vi "2022NewInstrumentationU6.vi"() -> ()   [LabVIEW 2021]
uses:
  <vilib>/Analysis/baseanly.llb/Mean (DBL).vi
  <vilib>/Analysis/NI_AALBase.lvlib
panel:
  out "ShuntCurrent":dbl[](graph)
  in  "Clear Charts Button":bool
  out "Runtank Weight":dbl(slide) scale=0.0..5.0
  out "Injector Pressure":dbl(knob) scale=700.0..800.0
  out "Runtank Pressure":dbl(knob) scale=700.0..800.0
  out "N2 Pressure":dbl(knob) scale=700.0..800.0
  out "N20 Pressure":dbl(knob) scale=700.0..800.0
  in  "Binary 2":bool
  in  "AIN Range":u16(ring) items=["LJ_rgBIP10V", "LJ_rgBIP1V", "LJ_rgBIPP1V", "LJ_rgBIPP01V"]
  in  "FirstFound":bool=TRUE
  in  "Address":string="1"
  out "Error Message 2":string="No Error"
  out "error out":errorcluster
  out "Cold Junction Temp":dbl=41420.0 format="%.6f"
  out "L-Thrust":dbl(graph)
  out "L-RunTank":dbl(graph)
  out "P-CombChamb - Deactivated":dbl[](graph)
  out "P-Injector":dbl(graph)
  out "T-PoComb":dbl(graph)
  out "T-CombCham":dbl(graph)
  out "T-Injector":dbl(graph)
  out "T-RunTank":dbl(graph)
  out "P-RunTank":dbl(graph)
  out "P-N2Flow":dbl(graph)
  out "P-N2OFlow":dbl(graph)
  in  "file name":string
  in  "file path":path
  in  "Iterations/Second":i32=1
  in  "Binary":bool
  in  "StreamSettlingFactor":i32
  in  "Resolution Index":u8
  in  "Range Constants":u8[](array[ring])=[0, 0, 0, 0] items=["LJ_rgBIP10V", "LJ_rgBIP1V", "LJ_rgBIPP1V", "LJ_rgBIPP01V"]
  out "Stream Parameters":T1 {"Device Backlog [%]" format="%.2f"}
  in  "PC buffer size (seconds)":dbl=10.0 format="%.2f"
  out "# of iterations":i32
  in  "Scan Rate (Hz)":dbl=1000.0 format="%.3f"
  in  "stop":bool
  out "Error Message":string
  # "Standard Test Parameters:"
  # "Range = 10\nResolution = 3\nSettling Factor = 2\nIterations/Second = 1\nScan Rate = 1300"
  # "This example streams from the first found USB U6."
  # "Data Output For Pressure, Temperature, and Load Sensors"
  # "The + scan list is the positive\nchannels.  For each element in\nthe + list, there must also be\nan element in the - list, which is\nthe negative channels.  For\nsingle-ended channels, put in\n199 for the negative channel.\n\nTo remove an element, right-click\non it, select Data Operations =>\nRemove Element.\n\nTo empty an array, right-click\nnear the edge, select Data\nOperations => Empty Array.\n\nOther useful operations:  From the\nOperate menu are \"Make Current\nValues Default\" and \"Reinitialize\nTo Default\"."
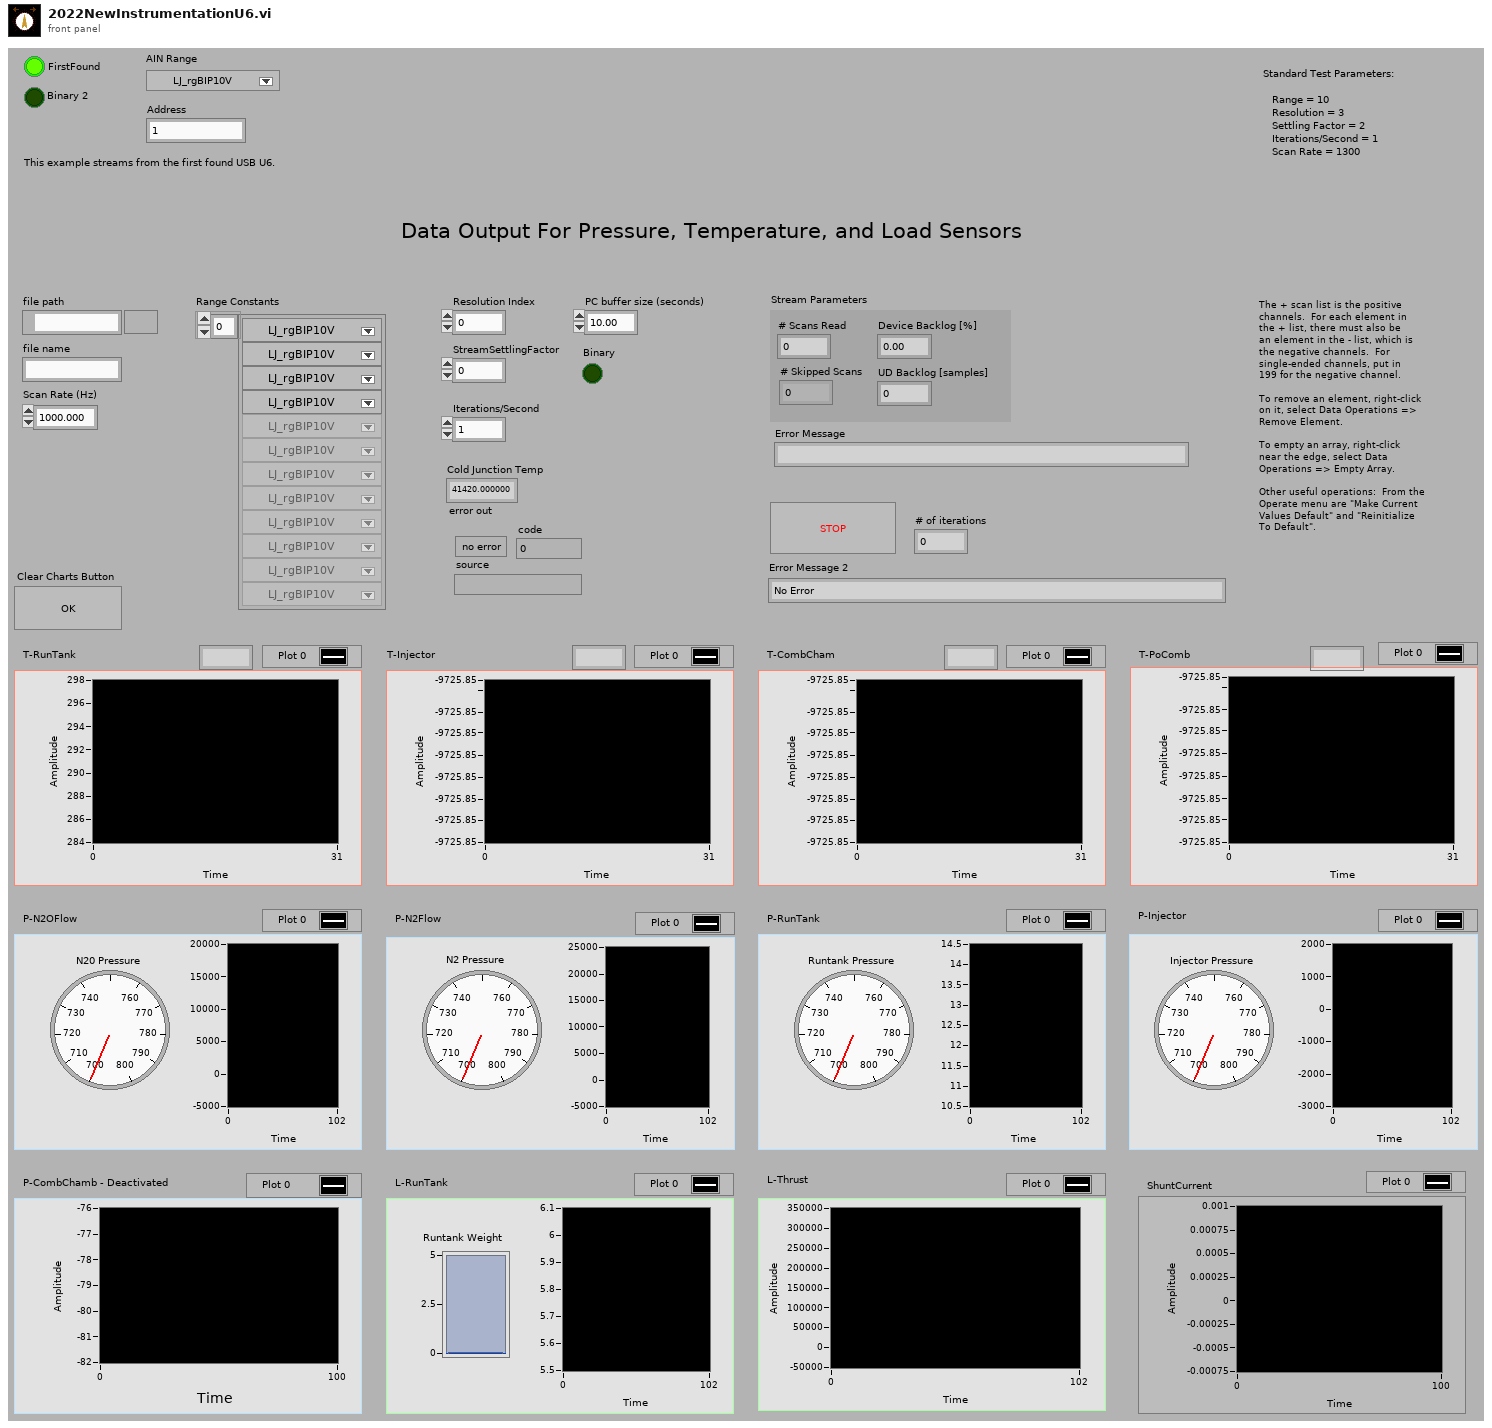
[diagram p1: front panel]
types:
  T1 = cluster{"# Scans Read":i32, "# Skipped Scans":i32, "Device Backlog [%]":dbl, "UD Backlog [samples]":i32}
  T2 = enum16{"open", "open or create", "create or replace", "create", "open (read-only)"}
  T3 = cluster{"PC buffer size (seconds)":dbl, "Resolution Index":u8, "StreamSettlingFactor":i32, "Binary":bool}
  T4 = typedef "Control 1.ctl" = dbl[][]
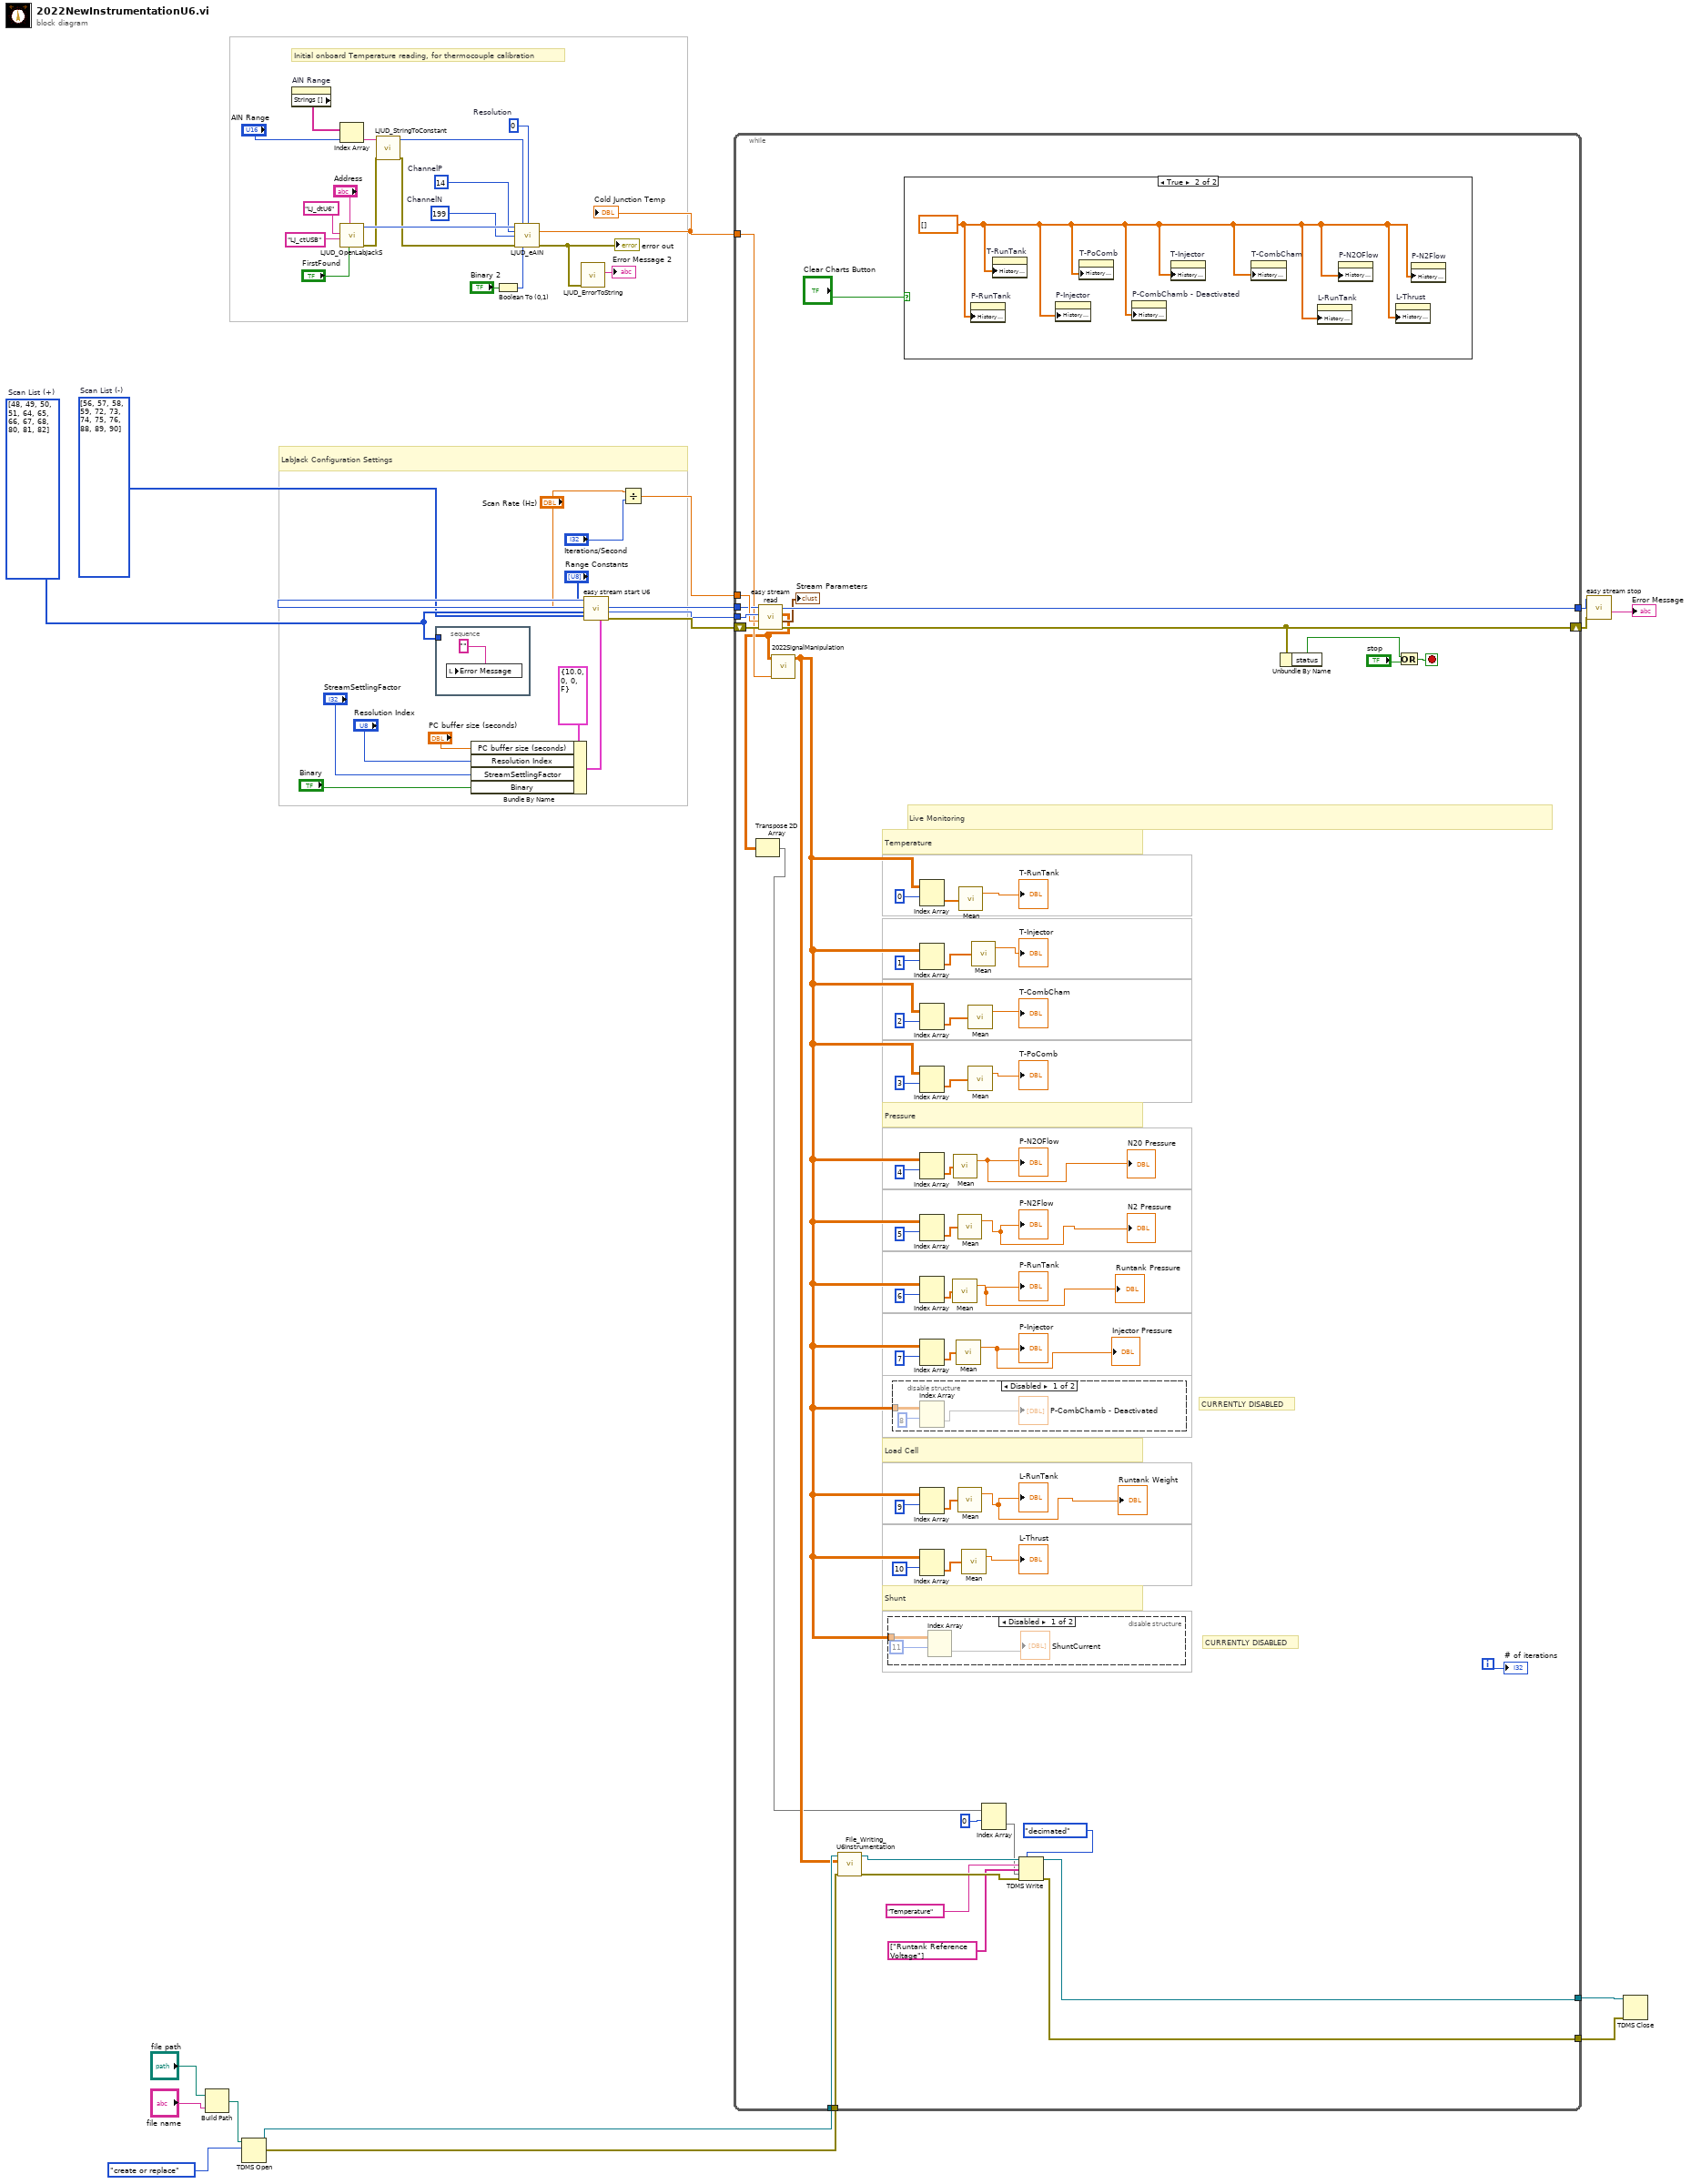
[diagram p0: block diagram]
diagram:
  w20 = 0  # Resolution
  w10 = 199  # ChannelN
  w11 = 14  # ChannelP
  w28 = u8[] [56, 57, 58, 59, 72, 73, 74, 75, 76, 88, 89, 90]  # Scan List (-)
  w29 = u8[] [48, 49, 50, 51, 64, 65, 66, 67, 68, 80, 81, 82]  # Scan List (+)
  # "LabJack Configuration Settings"
  # "Initial onboard Temperature reading, for thermocouple calibration"
  n1 = Build Path(base path="file path", name or relative path="file name") -> (appended path=w7:path)
  n2 = TDMS Open(10:T2."create or replace" ("operation (0:open)"), 11:w7) -> (0:w3:errorcluster, 3:w4:refnum<k34>)  [unwired: 5 in]
  n3 = property on="AIN Range" class="Ring (strict)"() -> ("Strings []"=w16:string[])  [unwired: 2 in, 2 out]
  n4 = Index Array(array=w16, index="AIN Range") -> (element=w14:string)
  n5 = call "LJUD_OpenLabJackS.vi"("FirstFound"="FirstFound", "Address"="Address", "ConnectionType"="LJ_ctUSB", "DeviceType"="LJ_dtU6") -> ("error out"=w19:errorcluster, "Handle"=w23:i32)  [unwired: 5 in, 1 out]
  n6 = call "LJUD_StringToConstant.vi"("error in"=w19, "String"=w14) -> ("error out"=w18:errorcluster, "Constant Number"=w21:i32)  [unwired: 8 in]
  n7 = stacked-sequence {
    tunnel: w29 -> [_]
    frame #0 {
      n8 = local write "Error Message"("" ("Error Message")) -> ()
    }
  }
  n9 = Bundle By Name(cluster=T3 {"PC buffer size (seconds)"=10.0, "Resolution Index"=0, "StreamSettlingFactor"=0, "Binary"=FALSE} ("Advanced"), "PC buffer size (seconds)"="PC buffer size (seconds)", "Resolution Index"="Resolution Index", "StreamSettlingFactor"="StreamSettlingFactor", "Binary"="Binary") -> (w36:T3)
  n10 = Boolean To (0,1)(Boolean="Binary 2") -> (0, 1=w12:i16)
  n11 = call "LJUD_eAIN.vi"("Handle In"=w23, "Range"=w21, "Resolution"=w20, "ChannelP"=w11, "ChannelN"=w10, "error in"=w18, "Binary"=w12) -> ("Voltage"=w6:dbl, "error out"=w26:errorcluster)  [unwired: 6 in, 1 out]
  "Cold Junction Temp" <- w6
  "error out" <- w26
  n12 = call "LJUD_ErrorToString.vi"("error in"=w26) -> ("String"=→"Error Message 2":string)  [unwired: 10 in]
  n13 = call "easy stream start U6.vi"("Advanced"=w36, "Scan List (-)"=w28, "Scan List (+)"=w29, "Scan Rate (Hz)"="Scan Rate (Hz)", "Range Constants"="Range Constants") -> ("error out"=w45:errorcluster, "# Channels"=w44:i32, "Handle Out"=w43:i32)  [unwired: 3 in, 1 out]
  n14 = Divide(x="Scan Rate (Hz)", y="Iterations/Second") -> (x/y=w40:dbl)
  n15 = while {
    tunnel: w43 -> [w93]
    tunnel: w44 -> [w100]
    shift-left: w45 -> [w101]
    shift-right: [w98] -> w42
    tunnel: w40 -> [w99]
    tunnel: [w97] -> w39
    tunnel: w6 -> [w90]
    tunnel: w4 -> [w87]
    tunnel: w3 -> [w86]
    tunnel: [w48] -> w2
    tunnel: [w47] -> w1
    i -> [w102]
    stop <- w103 stop-if-true
    # "CURRENTLY DISABLED"
    # "CURRENTLY DISABLED"
    # "Shunt"
    # "Load Cell"
    # "Pressure"
    # "Temperature"
    # "Live Monitoring"
    n16 = call "easy stream read.vi"("error in"=w101, "Scans To Read"=w99, "# Channels In Stream"=w100, "Handle In"=w93) -> ("error out"=w98:errorcluster, "Stream Parameters"=→"Stream Parameters":T1, "Data"=w85:dbl[][], "Handle Out"=w97:i32)  [unwired: 4 in]
    n17 = Transpose 2D Array(2D array=w85) -> (transposed array=w77:dbl[][])
    n18 = call "2022SignalManipulation.vi"("Cold Junction Temp 2"=w90, "Data"=w85) -> ("Output"=w84:T4)  [unwired: 9 in]
    n19 = call "File_Writing_U6Instrumentation.vi"("error in (no error)"=w86, "Output"=w84, "Refnum in"=w87) -> ("error out"=w81:errorcluster, "Refnum out"=w82:refnum<k34>)  [unwired: 7 in]
    n20 = disable-structure shown="Disabled" {
      disable-tunnel: w84 -> [w104 _]
      frame Disabled {
        n21 = Index Array(array=w104, index (row)=11) -> (element=→"ShuntCurrent":dbl[])  [unwired: 1 in]
      }
      frame Enabled {
      }
    }
    n22 = disable-structure shown="Disabled" {
      disable-tunnel: w84 -> [w107 _]
      frame Disabled {
        n23 = Index Array(array=w107, index (row)=8) -> (element=→"P-CombChamb - Deactivated":dbl[])  [unwired: 1 in]
      }
      frame Enabled {
      }
    }
    n24 = case shown="True" "Clear Charts Button" {
      frame False {
      }
      frame True {
        w110 = dbl[] []
        n25 = property on="P-RunTank" class="WFChart (strict)"("History Data"=w110) -> ()  [unwired: 2 in, 2 out]
        n26 = property on="T-RunTank" class="WFChart (strict)"("History Data"=w110) -> ()  [unwired: 2 in, 2 out]
        n27 = property on="P-Injector" class="WFChart (strict)"("History Data"=w110) -> ()  [unwired: 2 in, 2 out]
        n28 = property on="T-PoComb" class="WFChart (strict)"("History Data"=w110) -> ()  [unwired: 2 in, 2 out]
        n29 = property on="P-CombChamb - Deactivated" class="WFChart (strict)"("History Data"=w110) -> ()  [unwired: 2 in, 2 out]
        n30 = property on="T-Injector" class="WFChart (strict)"("History Data"=w110) -> ()  [unwired: 2 in, 2 out]
        n31 = property on="T-CombCham" class="WFChart (strict)"("History Data"=w110) -> ()  [unwired: 2 in, 2 out]
        n32 = property on="L-RunTank" class="WFChart (strict)"("History Data"=w110) -> ()  [unwired: 2 in, 2 out]
        n33 = property on="P-N2OFlow" class="WFChart (strict)"("History Data"=w110) -> ()  [unwired: 2 in, 2 out]
        n34 = property on="L-Thrust" class="WFChart (strict)"("History Data"=w110) -> ()  [unwired: 2 in, 2 out]
        n35 = property on="P-N2Flow" class="WFChart (strict)"("History Data"=w110) -> ()  [unwired: 2 in, 2 out]
      }
    }
    n36 = Index Array(array=w84, index (row)=0) -> (element=w89:dbl[])  [unwired: 1 in]
    n37 = Index Array(array=w84, index (row)=1) -> (element=w67:dbl[])  [unwired: 1 in]
    n38 = Index Array(array=w84, index (row)=2) -> (element=w65:dbl[])  [unwired: 1 in]
    n39 = Index Array(array=w84, index (row)=3) -> (element=w63:dbl[])  [unwired: 1 in]
    n40 = Index Array(array=w84, index (row)=4) -> (element=w61:dbl[])  [unwired: 1 in]
    n41 = Index Array(array=w84, index (row)=5) -> (element=w59:dbl[])  [unwired: 1 in]
    n42 = Index Array(array=w84, index (row)=6) -> (element=w57:dbl[])  [unwired: 1 in]
    n43 = Index Array(array=w84, index (row)=7) -> (element=w55:dbl[])  [unwired: 1 in]
    n44 = Index Array(array=w84, index (row)=9) -> (element=w53:dbl[])  [unwired: 1 in]
    n45 = Index Array(array=w84, index (row)=10) -> (element=w51:dbl[])  [unwired: 1 in]
    n46 = call-poly <vilib>:"Mean.vi"("X"=w57) -> ("mean"=→"P-RunTank" →"Runtank Pressure":dbl)  [unwired: 1 out]
    n47 = call-poly <vilib>:"Mean.vi"("X"=w61) -> ("mean"=→"P-N2OFlow" →"N20 Pressure":dbl)  [unwired: 1 out]
    n48 = call-poly <vilib>:"Mean.vi"("X"=w55) -> ("mean"=→"P-Injector" →"Injector Pressure":dbl)  [unwired: 1 out]
    n49 = call-poly <vilib>:"Mean.vi"("X"=w59) -> ("mean"=→"P-N2Flow" →"N2 Pressure":dbl)  [unwired: 1 out]
    n50 = call-poly <vilib>:"Mean.vi"("X"=w53) -> ("mean"=→"L-RunTank" →"Runtank Weight":dbl)  [unwired: 1 out]
    n51 = call-poly <vilib>:"Mean.vi"("X"=w89) -> ("mean"=→"T-RunTank":dbl)  [unwired: 1 out]
    n52 = call-poly <vilib>:"Mean.vi"("X"=w51) -> ("mean"=→"L-Thrust":dbl)  [unwired: 1 out]
    n53 = call-poly <vilib>:"Mean.vi"("X"=w65) -> ("mean"=→"T-CombCham":dbl)  [unwired: 1 out]
    n54 = call-poly <vilib>:"Mean.vi"("X"=w63) -> ("mean"=→"T-PoComb":dbl)  [unwired: 1 out]
    n55 = call-poly <vilib>:"Mean.vi"("X"=w67) -> ("mean"=→"T-Injector":dbl)  [unwired: 1 out]
    n56 = Index Array(array=w77, index (row)=0) -> (element=w78:dbl[])  [unwired: 1 in]
    n57 = TDMS Write(0:w82, 1:enum16{"decimated", "interleaved"}."decimated" ("data layout (0:decimated)"), 5:"Temperature" ("group name in (Untitled)"), 7:string[] ["Runtank Reference Voltage"] ("channel name(s) in (Untitled)"), 9:w78, 11:w81) -> (4:w47:refnum<k34>, 15:w48:errorcluster)  [unwired: 2 out]
    n58 = Unbundle By Name(w98) -> ("status"=w95:bool)
    n59 = Or(x=w95, y="stop") -> (x .or. y?=w103:bool)
    "# of iterations" <- w102
  }
  n60 = call "easy stream stop.vi"("error in"=w42, "Handle In"=w39) -> ("Error Message"=→"Error Message":string)  [unwired: 7 in, 2 out]
  n61 = TDMS Close(8:w2, 11:w1) -> ()  [unwired: 2 out]
